vi "practice1.vi"() -> ()   [LabVIEW 2020]
panel:
  in  "Vertical Scrollbar Visibility":T1(ring)
  in  "Horizontal Scrollbar Visibility":T1(ring)
  in  "error in":errorcluster
  out "error out":errorcluster
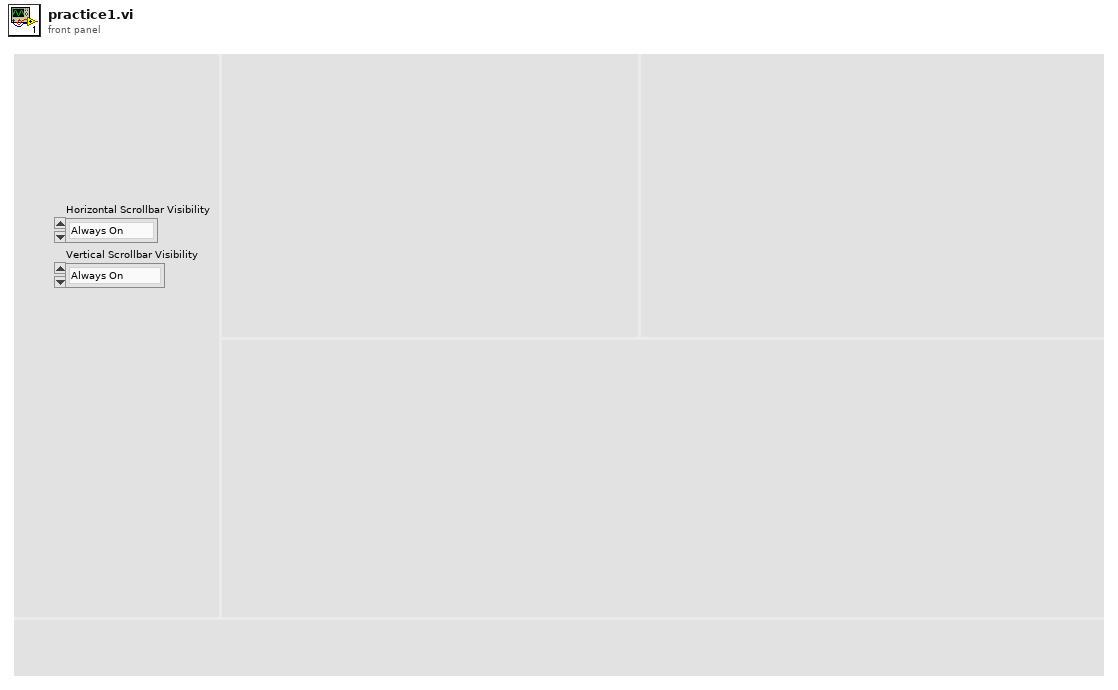
[diagram p1: front panel]
types:
  T1 = enum16{"Always On", "Always Off", "Off While Running"}
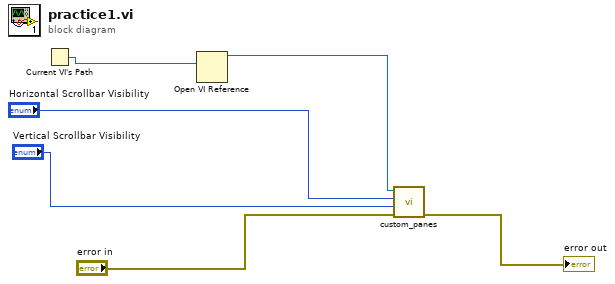
[diagram p0: block diagram]
diagram:
  n1 = Current VI's Path() -> (path=w1:path)
  n2 = Open VI Reference(vi path=w1) -> (vi reference=w2:refnum<vi>)  [unwired: 5 in, 1 out]
  n3 = call "custom_panes.vi"("error in"="error in", "Vertical Scrollbar Visibility"="Vertical Scrollbar Visibility", "Horizontal Scrollbar Visibility"="Horizontal Scrollbar Visibility", "reference"=w2) -> ("error out"=→"error out":errorcluster)  [unwired: 7 in]
